vi "_TCP Msg Write.vi"(8 "error in (no error)":errorcluster, 9 "Data Stream":string, 10 "Message Type":string, 11 "connection ID":refnum<k5>) -> (0 "error out":errorcluster, 1 "Packet":string, 2 "Checksum":u16, 3 "connection ID out":refnum<k5>)   [LabVIEW 2015]
doc: "Writes a package of data to a remote computer via TCP/IP. The VI appends an ID number to each packet. This ID number is used by the Comm TCP Read VI to parse the packet using the meta data. This technique allows appending variable name and type to each packet for ease of use while minimizing the transmission overhead.\n\nThe data must be passed in as a String. The user is responsible for casting or flattening the desired data into a String before passing it to this VI. \n\n* Use the same method for converting to/from String on both the Read and Write functions. For example, if you use the 'Cast' primitive to convert the data into a String, make sure that the 'Cast' primitive is used on the receiving side to convert the data from String to its original form."
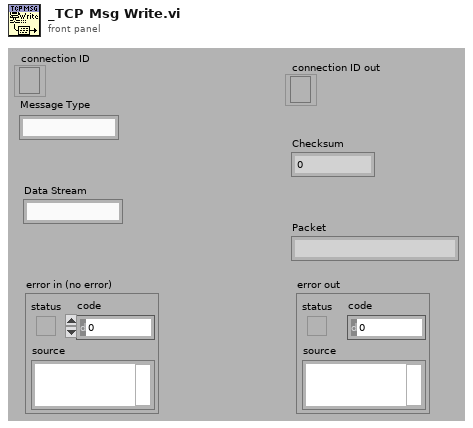
[diagram p1: front panel]
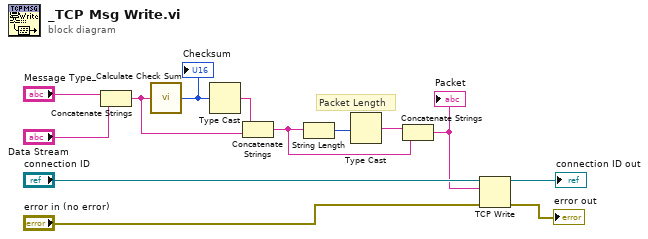
[diagram p0: block diagram]
diagram:
  # "Packet Length"
  n1 = Concatenate Strings("Message Type", "Data Stream") -> (w2:string)
  n2 = call "_Calculate Check Sum.vi"("Stream"=w2) -> ("Checksum"=w4:u16)
  "Checksum" <- w4
  n3 = Type Cast(x=w4) -> (*(type *) &x=w3:string)  [unwired: 1 out]
  n4 = Concatenate Strings(w3, w2) -> (w1:string)
  n5 = String Length(string=w1) -> (length=w8:i32)
  n6 = Type Cast(x=w8) -> (*(type *) &x=w7:string)  [unwired: 1 out]
  n7 = Concatenate Strings(w7, w1) -> (w6:string)
  "Packet" <- w6
  n8 = TCP Write(connection ID="connection ID", data in=w6, error in (no error)="error in (no error)") -> (connection ID out=→"connection ID out":refnum<k5>, error out=→"error out":errorcluster)  [unwired: 2 out]
